vi "DSF.Engine.Buffer Converter.Create.vi"(8 "error in (no error)":errorcluster, 10 "buffer channel count (1M)":i32=1000000, 11 "Buffer Converter type":refnum<class "Buffer Converter.lvclass">) -> (0 "error out":errorcluster, 3 "Buffer Converter":refnum<class "Buffer Converter.lvclass">)   [LabVIEW 2017, in "DSF.Engine.lvlib" / "Buffer Converter.lvclass"]
uses:
  Buffer Converter.lvclass
  Buffer Converter.lvclass/Buffer Converter.ctl
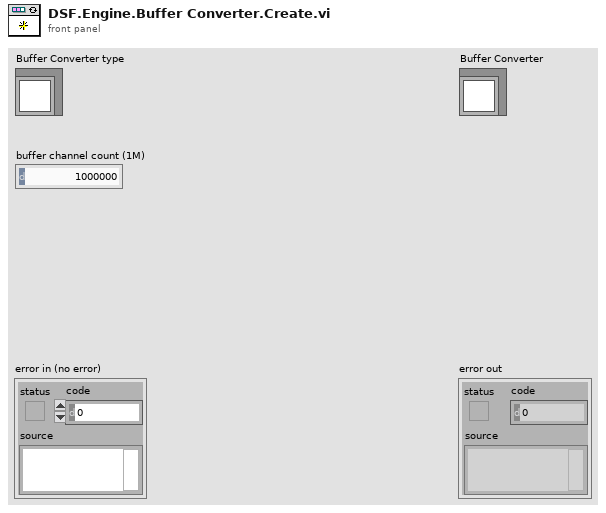
[diagram p1: front panel]
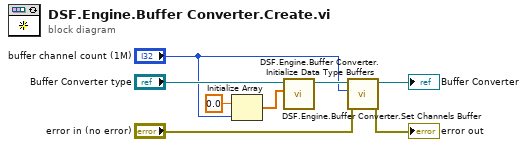
[diagram p0: block diagram]
diagram:
  n1 = Initialize Array(0.0 ("element"), "buffer channel count (1M)") -> (w6:dbl[])
  n2 = call "DSF.Engine.Buffer Converter.Set Channels Buffer.vi"("channels buffer"=w6, "Buffer Converter in"="Buffer Converter type") -> ("Buffer Converter out"=w4:refnum<class "Buffer Converter.lvclass">)  [unwired: 9 in]
  n3 = call "DSF.Engine.Buffer Converter.Initialize Data Type Buffers.vi"("error in (no error)"="error in (no error)", "channel count (1M)"="buffer channel count (1M)", "Buffer Converter in"=w4) -> ("error out"=→"error out":errorcluster, "Buffer Converter out"=→"Buffer Converter":refnum<class "Buffer Converter.lvclass">)  [unwired: 7 in]
